vi "Change List Type.vi"(8 "error in (no error)":errorcluster, 10 "List type":T1 caption="HLP_Format Code List Type", 11 "Numeric Data Type in":refnum<class "Numeric Data Type.lvclass">) -> (0 "error out":errorcluster, 3 "Numeric Data Type out":refnum<class "Numeric Data Type.lvclass">)   [LabVIEW 2018, in "Numeric Data Type.lvclass"]
uses:
  Numeric Data Type.lvclass
  Format Code Type List Enum.ctl
  <vilib>/Utility/miscctls.llb/LVRowAndColumnUnsignedTypeDef.ctl
  Reference List Type.vi
  Reference Format Codes.vi
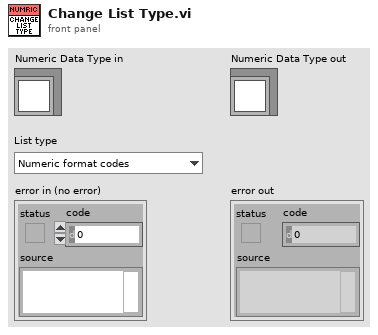
[diagram p1: front panel]
types:
  T1 = typedef "Numeric Data Type.lvclass/Format Code Type List Enum.ctl" = enum16{"Numeric format codes", "Relative time format codes", "Absolute time format codes"}
  T2 = typedef "LVRowAndColumnUnsignedTypeDef.ctl" = cluster{"Row":u32, "Column":u32}
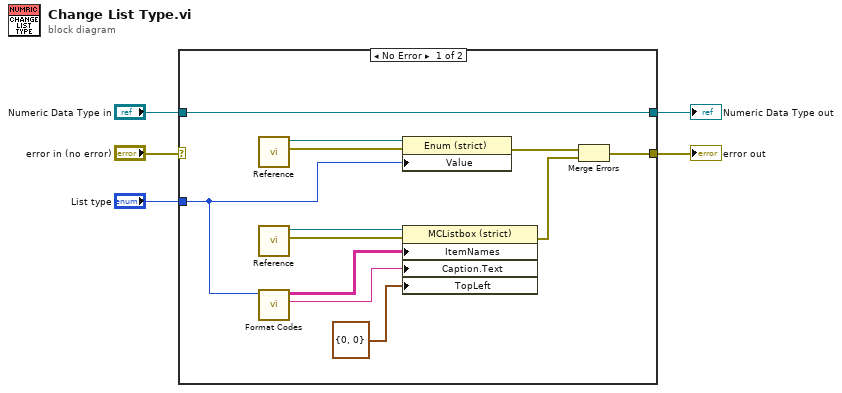
[diagram p0: block diagram]
diagram:
  n1 = case shown="No Error" "error in (no error)" {
    selector: "error in (no error)" -> [_ w19]
    tunnel: [w10 w19] -> w4
    tunnel: [w17 w18] -> w2
    tunnel: "Numeric Data Type in" -> [w17 w18]
    tunnel: "List type" -> [w16 _]
    frame No Error {
      n2 = call-poly "Reference.vi"() -> ("error out"=w8:errorcluster, "List Type"=w9:refnum<vi>)  [unwired: 10 in]
      n3 = call-poly "Reference.vi"() -> ("error out"=w6:errorcluster, "Format Codes"=w7:refnum<vi>)  [unwired: 10 in]
      n4 = call "Format Codes.vi"("List type"=w16) -> ("Caption"=w14:string, "Item Names"=w15:string[][])  [unwired: 9 in]
      n5 = property class="Enum (strict)"(reference=w9, error in=w8, "Value"=w16) -> (error out=w12:errorcluster)  [unwired: 1 out]
      n6 = property on="Property Node" class="MCListbox (strict)"(reference=w7, error in=w6, "ItemNames"=w15, "Caption.Text"=w14, "TopLeft"=T2 {"Row"=0, "Column"=0} ("Top Left Visible Cell")) -> (error out=w11:errorcluster)  [unwired: 1 out]
      n7 = Merge Errors(w12, w11) -> (w10:errorcluster)
    }
    frame Error {
    }
  }
  "error out" <- w4
  "Numeric Data Type out" <- w2
